vi "Process Hardware Compare Data.vi"() -> ()   [LabVIEW 2013]
uses:
  Ctrls/ReadInfo.ctl
panel:
  out "error out":errorcluster
  in  "error in (no error)":errorcluster
  in  "Compare Bits Out":T1[](array[typedef]) {"Expected Value(s)" format="%.0x"}
  in  "Error Locations":dbl[](array[numeric]) caption="sample numbers"
  out "Parity Error":bool
  out "MIPI Data Read from DUT":cluster{"Read Data":u8[]}[](array[cluster])=[{"Read Data"=[1]}] {"Read Data" format="%.0x"}
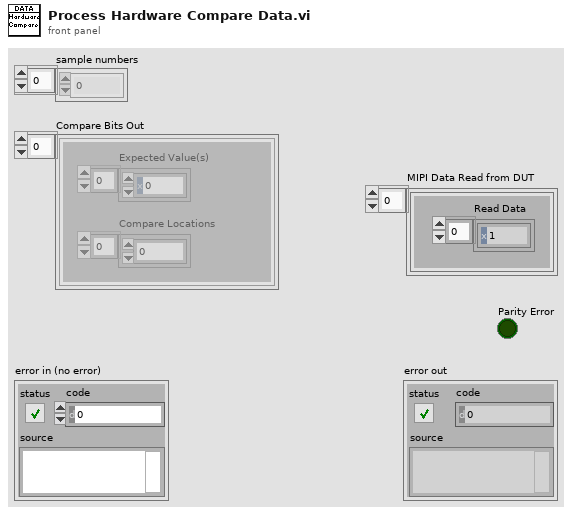
[diagram p1: front panel]
types:
  T1 = typedef "ReadInfo.ctl" = cluster{"Expected Value(s)":u8[], "Compare Locations":u32[]}
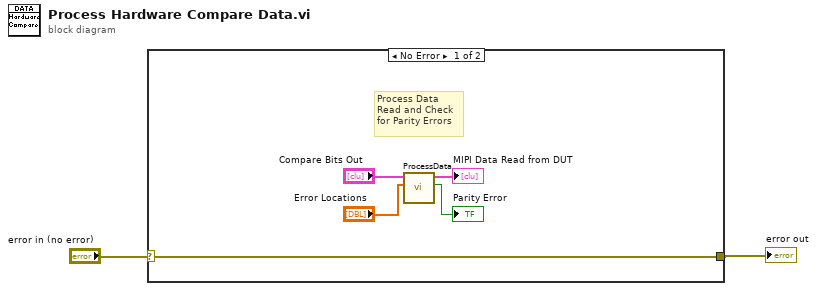
[diagram p0: block diagram]
diagram:
  n1 = case shown="No Error" "error in (no error)" {
    selector: "error in (no error)" -> [w7 w8]
    tunnel: [w7 w8] -> w1
    frame No Error {
      # "Process Data Read and Check for Parity Errors"
      n2 = call "ProcessData.vi"("Error Loacations"="Error Locations", "Read Info"="Compare Bits Out") -> ("Parity Error"=→"Parity Error":bool, "Read MIPI Data"=→"MIPI Data Read from DUT":cluster{"Read Data":u8[]}[])  [unwired: 8 in]
    }
    frame Error {
    }
  }
  "error out" <- w1
